vi "ProdaNG.WriteToFile.vi"(6 "append (F)":bool, 8 "error in":errorcluster, 9 "header":string, 10 "addition":string, 11 "file":path) -> (0 "error out":errorcluster)   [LabVIEW 2016]
doc: "Writes to a file.\nIf <B>append</B> is false (default), the file will be rewritten.\nIf <B>append</B> is true, the new data will be appended to the file.\nSupports a <B>header</B> line which will be placed on top of the file when it is created or rewritten. This <B>header</B> line requires a newline at the end."
panel:
  # "Added at begin only if file is created"
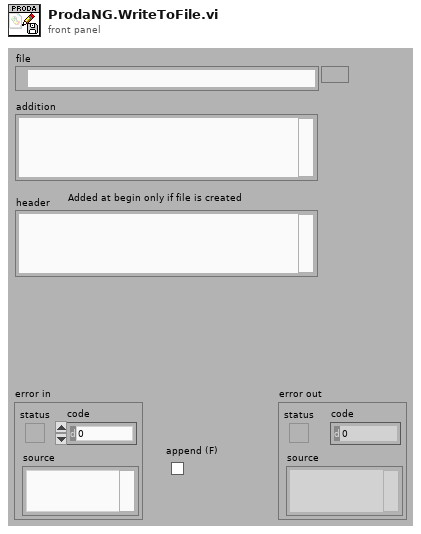
[diagram p1: front panel]
types:
  T1 = enum16{"deny read/write", "deny write-only", "deny none"}
  T2 = enum16{"open", "replace", "create", "open or create", "replace or create", "replace or create with confirmation"}
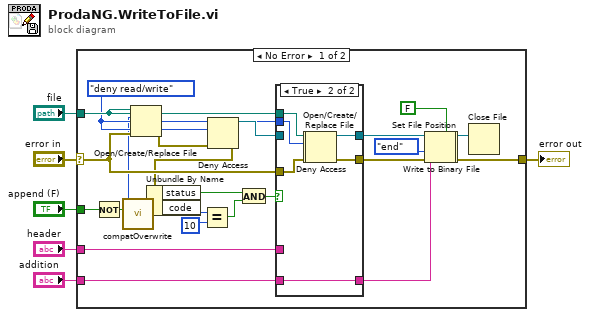
[diagram p0: block diagram]
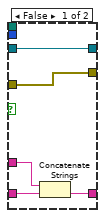
[diagram p2: hidden frame]
diagram:
  n1 = case shown="No Error" "error in" {
    selector: "error in" -> [w21 w46]
    tunnel: [w14 w46] -> w6
    tunnel: "append (F)" -> [w30 _]
    tunnel: "file" -> [w28 _]
    tunnel: "addition" -> [w23 _]
    tunnel: "header" -> [w25 _]
    frame No Error {
      w15 = T1."deny read/write" ("deny mode (2)")
      n2 = Not(x=w30) -> (.not. x?=w24:bool)
      n3 = call <vilib>:"compatOverwrite.vi"("overwrite (F)"=w24) -> ("overwrite?"=w9:T2)
      n4 = Open/Create/Replace File(file path (use dialog)=w28, error in=w21, operation (0:open)=w9) -> (refnum out=w10:refnum<file>, error out=w7:errorcluster)  [unwired: 4 out]
      n5 = Deny Access(4:w7, 6:w15, 7:w10) -> (0:w8:errorcluster, 3:w27:refnum<file>)
      n6 = Unbundle By Name(w8) -> ("status"=w17:bool, "code"=w20:i32)
      n7 = Equal?(x=w20, y=10) -> (x = y?=w18:bool)
      n8 = And(x=w17, y=w18) -> (x .and. y?=w16:bool)
      n9 = case shown="True" w16 {
        tunnel: [w33 w45] -> w29
        tunnel: w28 -> [_ w44]
        tunnel: w27 -> [w37 _]
        tunnel: [w37 w43] -> w26
        tunnel: w25 -> [w35 _]
        tunnel: [w34 w42] -> w22
        tunnel: w23 -> [w36 w42]
        tunnel: w21 -> [w33 w41]
        tunnel: w15 -> [_ w40]
        frame False {
          n10 = Concatenate Strings(w35, w36) -> (w34:string)
        }
        frame True {
          n11 = Open/Create/Replace File(file path (use dialog)=w44, error in=w41) -> (refnum out=w38:refnum<file>, error out=w39:errorcluster)  [unwired: 5 out]
          n12 = Deny Access(4:w39, 6:w40, 7:w38) -> (0:w45:errorcluster, 3:w43:refnum<file>)
        }
      }
      n13 = Set File Position(refnum=w26, from (0:start)=enum16{"start", "end", "current"}."end" ("pos mode (0:2)"), error in=w29) -> (refnum out=w13:refnum<file>, error out=w12:errorcluster)  [unwired: 1 out]
      n14 = Write to Binary File(file (use dialog)=w13, data=w22, error in=w12, 5:FALSE ("prepend array or string size? (T)")) -> (refnum out=w32:refnum<file>, error out=w14:errorcluster)  [unwired: 3 out]
      n15 = Close File(refnum=w32) -> ()  [unwired: 1 in, 2 out]
    }
    frame Error {
    }
  }
  "error out" <- w6
